vi "Earliest PageSelector Page.vi"(8 "error in (no error)":errorcluster, 11 "PageSelector ref in":refnum<vi>) -> (0 "error out":errorcluster, 2 "PageSelector":T1, 3 "PageSelector ref out":refnum<vi>)   [LabVIEW 2019]
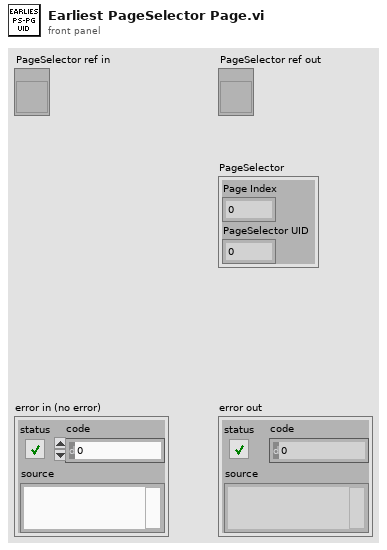
[diagram p1: front panel]
types:
  T1 = cluster{"Page Index":i32, "PageSelector UID":i32}
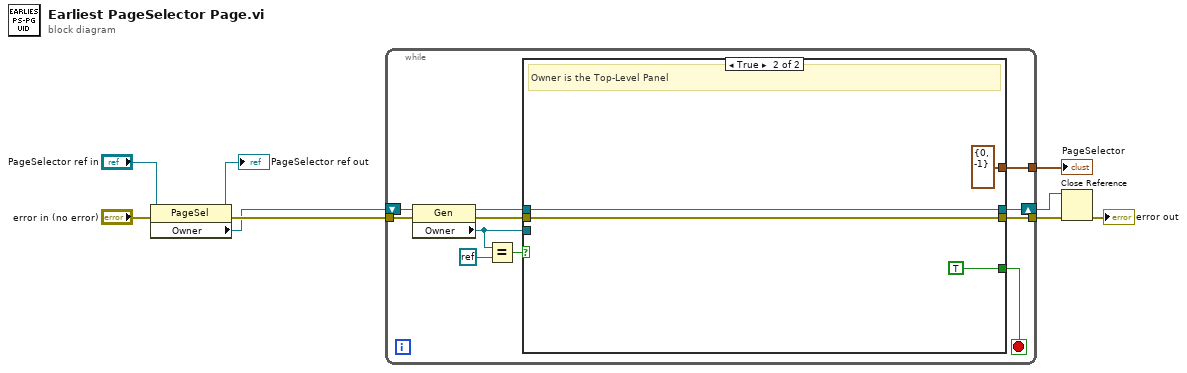
[diagram p0: block diagram]
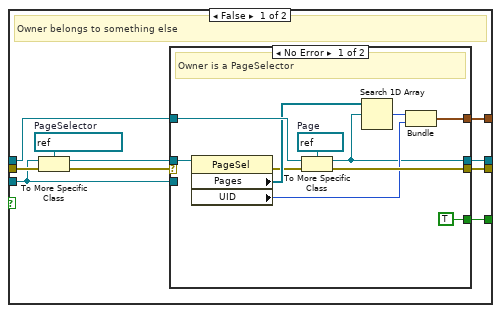
[diagram p2: hidden frame]
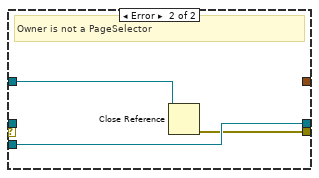
[diagram p3: hidden frame]
diagram:
  n1 = property class="PageSel"(reference="PageSelector ref in", error in="error in (no error)") -> (reference out=→"PageSelector ref out":refnum<vi>, error out=w6:errorcluster, "Owner"=w5:refnum<vi>)
  n2 = while {
    tunnel: w6 -> [w17]
    shift-right: [w15] -> w3
    shift-left: w5 -> [w18]
    tunnel: [w11] -> w4
    tunnel: [w10] -> w1
    stop <- w16 stop-if-true
    n3 = property class="Gen"(reference=w18, error in=w17) -> (reference out=w12:refnum<vi>, error out=w13:errorcluster, "Owner"=w14:refnum<vi>)
    n4 = Equal?(x=w14, y=refnum<k0> refnum) -> (x = y?=w19:bool)
    n5 = case shown="True" w19 {
      tunnel: [w27 TRUE ("Boolean")] -> w16
      tunnel: [w25 w46] -> w15
      tunnel: w14 -> [w26 _]
      tunnel: w13 -> [w29 w47]
      tunnel: w12 -> [w24 w46]
      tunnel: [w23 w47] -> w11
      tunnel: [w21 cluster{"index of element":i32, "UID":i32} {"index of element"=0, "UID"=-1}] -> w10
      frame False {
        w30 = refnum<vi> refnum  # PageSelector
        # "Owner belongs to something else"
        n6 = To More Specific Class(target class=w30, reference=w26, error in=w29) -> (specific class reference=w22:refnum<vi>, error out=w28:errorcluster)
        n7 = case shown="No Error" w28 {
          tunnel: [TRUE ("Boolean") _] -> w27
          tunnel: w26 -> [_ w44]
          tunnel: [w31 w44] -> w25
          tunnel: w24 -> [w38 w43]
          tunnel: [w39 w42] -> w23
          tunnel: w22 -> [w37 _]
          tunnel: [w32 _] -> w21
          frame No Error {
            w40 = refnum<vi> refnum  # Page
            # "Owner is a PageSelector"
            n8 = property class="PageSel"(reference=w37) -> (error out=w35:errorcluster, "Pages"=w36:refnum<vi>[], "UID"=w33:i32)  [unwired: 1 in, 1 out]
            n9 = To More Specific Class(target class=w40, reference=w38, error in=w35) -> (specific class reference=w31:refnum<vi>, error out=w39:errorcluster)
            n10 = Search 1D Array(1D array=w36, element=w31) -> (index of element=w34:i32)  [unwired: 1 in]
            n11 = Bundle("index of element"=w34, "UID"=w33) -> (w32:cluster{"index of element":i32, "UID":i32})  [unwired: 1 in]
          }
          frame Error {
            # "Owner is not a PageSelector"
            n12 = Close Reference(reference=w43) -> (error out=w42:errorcluster)  [unwired: 1 in]
          }
        }
      }
      frame True {
        # "Owner is the Top-Level Panel"
      }
    }
  }
  "PageSelector" <- w1
  n13 = Close Reference(reference=w3, error in (no error)=w4) -> (error out=→"error out":errorcluster)
